vi "脑钱包-字符-地址与私钥.vi"(8 "error in (no error)":cluster{"状态":bool, "代码":i32, "源":string} caption="错误输入（无错误）", 11 "脑字符":string="str1") -> (0 "error out":cluster{"状态":bool, "代码":i32, "源":string} caption="错误输出", 2 "私钥":string, 3 "地址":string)   [LabVIEW 2020]
uses:
  C:/Program Files (x86)/National Instruments/LabVIEW 2020/examples/Connectivity/Python/support/PythonVersionsEnum.ctl
panel:
  in  "Python版本":T1=enum."3.6"
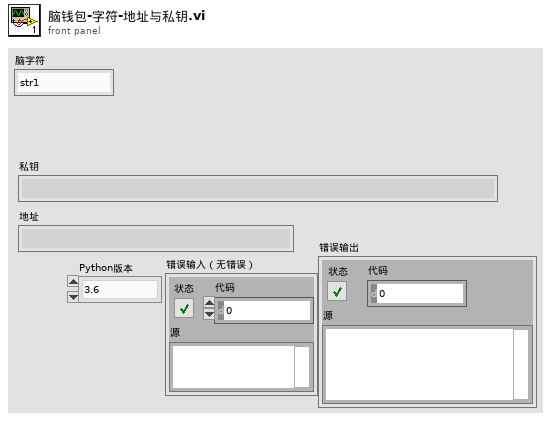
[diagram p1: front panel]
types:
  T1 = typedef "PythonVersionsEnum.ctl" = enum16{"2.7", "3.6"}
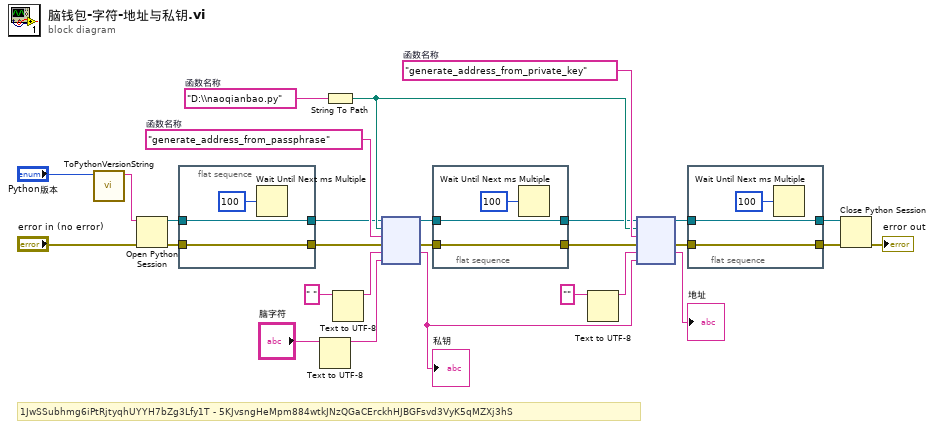
[diagram p0: block diagram]
diagram:
  w21 = "generate_address_from_private_key"  # 函数名称
  w24 = "generate_address_from_passphrase"  # 函数名称
  w25 = "D:\\naoqianbao.py"  # 函数名称
  # "1JwSSubhmg6iPtRjtyqhUYYH7bZg3Lfy1T - 5KJvsngHeMpm884wtkJNzQGaCErckhHJBGFsvd3VyK5qMZXj3hS"
  n1 = call "ToPythonVersionString.vi"("Python版本"="Python版本") -> ("python版本字符串"=w28:string)  [unwired: 10 in]
  n2 = Open Python Session(python version=w28, 3:"error in (no error)") -> (session out=w16:refnum<k35>, error out=w6:errorcluster)  [unwired: 1 in]
  n3 = flat-sequence {
    tunnel: w16 -> [w30]
    tunnel: [w30] -> w15
    tunnel: [w29] -> w5
    tunnel: w6 -> [w29]
    frame #0 {
      n4 = Wait Until Next ms Multiple(millisecond multiple=u32 100 ("毫秒倍数")) -> ()  [unwired: 1 out]
    }
  }
  n5 = Text to UTF-8(11:"脑字符") -> (3:w22:string)  [unwired: 2 in, 1 out]
  n6 = String To Path(string=w25) -> (path=w17:path)
  n7 = Text to UTF-8(11:" ") -> (3:w20:string)  [unwired: 2 in, 1 out]
  n8 = node(w15, w17, w24, w5, w20, w22) -> (w14:refnum<k35>, w4:errorcluster, w19:string)  [unwired: 1 in, 2 out]
  "私钥" <- w19
  n9 = flat-sequence {
    tunnel: w14 -> [w33]
    tunnel: [w33] -> w13
    tunnel: [w32] -> w3
    tunnel: w4 -> [w32]
    frame #0 {
      n10 = Wait Until Next ms Multiple(millisecond multiple=u32 100 ("毫秒倍数")) -> ()  [unwired: 1 out]
    }
  }
  n11 = Text to UTF-8(11:"") -> (3:w7:string)  [unwired: 2 in, 1 out]
  n12 = node(w13, w17, w21, w3, w7, w19) -> (w10:refnum<k35>, w1:errorcluster, →"地址":string)  [unwired: 1 in, 2 out]
  n13 = flat-sequence {
    tunnel: [w36] -> w9
    tunnel: w10 -> [w36]
    tunnel: [w35] -> w2
    tunnel: w1 -> [w35]
    frame #0 {
      n14 = Wait Until Next ms Multiple(millisecond multiple=u32 100 ("毫秒倍数")) -> ()  [unwired: 1 out]
    }
  }
  n15 = Close Python Session(session in=w9, error in=w2) -> (11:→"error out":errorcluster)
